vi "Display Features.vi"(6 "Local Data in":T2, 7 "UI References":T1, 8 "error in (no error)":errorcluster, 10 "Action":enum16{"All", "Preview", "Image"}(ring)=enum."Image") -> (0 "error out":errorcluster, 4 "Local Data out":T2)   [LabVIEW 2024]
uses:
  Controls/RVHR - Local Data.ctl
  Controls/Test Cluster.ctl
  Controls/Excluded Information.ctl
  Controls/Language.ctl
  Controls/Device_Type.ctl
  <vilib>/Utility/miscctls.llb/LVRectTypeDef.ctl
  <vilib>/Utility/miscctls.llb/LVBoundsTypeDef.ctl
  Controls/RVHR - UI Refs.ctl
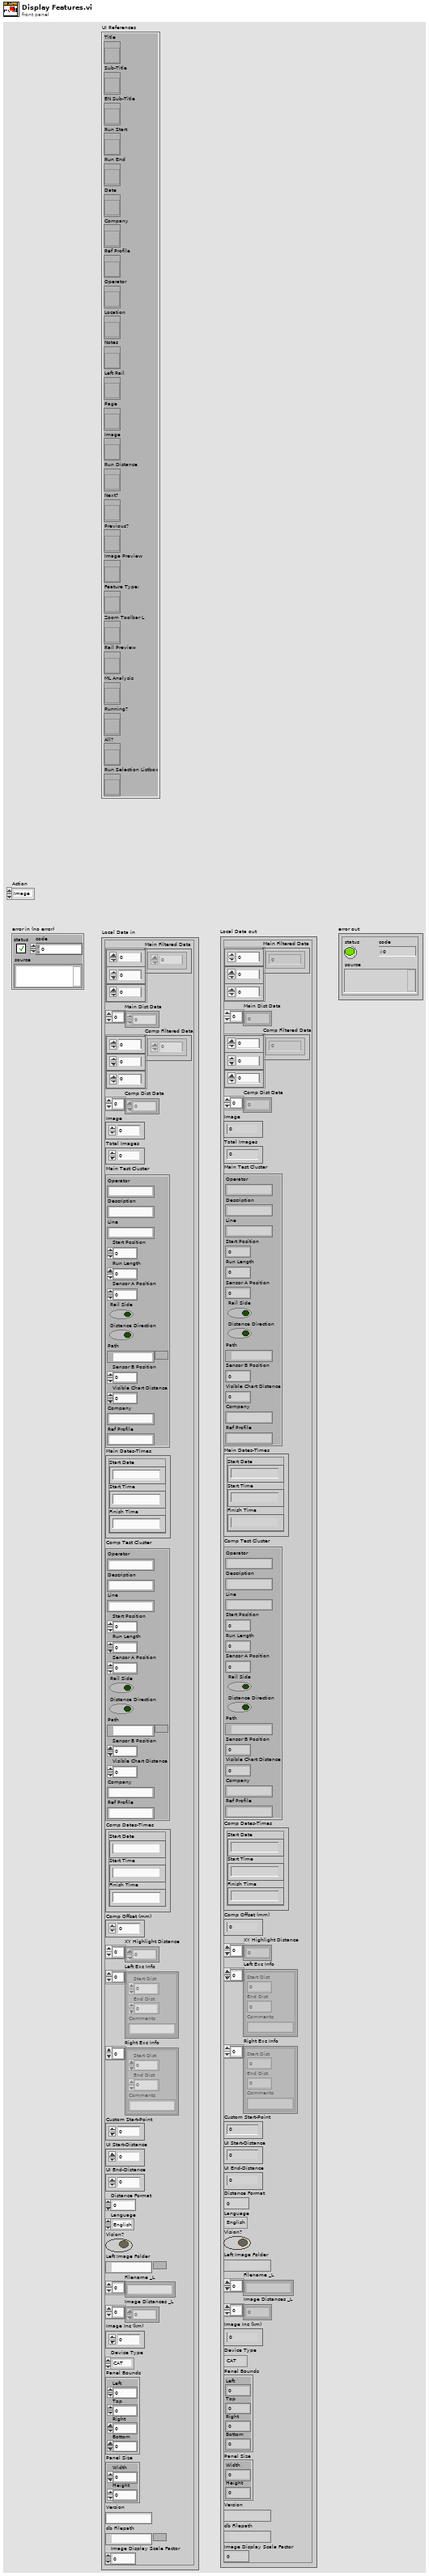
[diagram p1: front panel]
types:
  T1 = typedef "RVHR - UI Refs.ctl" = cluster{"Title":refnum<vi>, "Sub-Title":refnum<vi>, "EN Sub-Title":refnum<vi>, "Run Start":refnum<vi>, "Run End":refnum<vi>, "Date":refnum<vi>, "Company":refnum<vi>, "Ref Profile":refnum<vi>, "Operator":refnum<vi>, "Location":refnum<vi>, "Notes":refnum<vi>, "Left Rail":refnum<vi>, "Page":refnum<vi>, "Image":refnum<vi>, "Run Distance":refnum<vi>, "Next?":refnum<vi>, "Previous?":refnum<vi>, "Image Preview":refnum<vi>, "Feature Type:":refnum<vi>, "Zoom Toolbar L":refnum<vi>, "Rail Preview":refnum<vi>, "ML Analysis":refnum<vi>, "Running?":refnum<vi>, "All?":refnum<vi>, "Run Selection Listbox":refnum<vi>}
  T2 = typedef "RVHR - Local Data.ctl" = cluster{"Main Filtered Data":dbl[][][], "Main Dist Data":dbl[], "Comp Filtered Data":dbl[][][], "Comp Dist Data":dbl[], "Image":u16, "Total Images":u16, "Main Test Cluster":T3, "Main Dates-Times":cluster{"Start Date":string, "Start Time":string, "Finish Time":string}, "Comp Test Cluster":T3, "Comp Dates-Times":cluster{"Start Date":string, "Start Time":string, "Finish Time":string}, "Comp Offset (mm)":i64, "XY Highlight Distance":dbl[], "Left Exc Info":T4[], "Right Exc Info":T4[], "Custom Start-Point":dbl, "UI Start-Distance":dbl, "UI End-Distance":dbl, "Distance Format":u8, "Language":T5, "Vision?":bool, "Left Image Folder":path, "Filename _L":string[], "Image Distances _L":dbl[], "Image Inc (km)":dbl, "Device Type":T6, "Panel Bounds":T7, "Panel Size":T8, "Version":string, "db Filepath":path, "Image Display Scale Factor":dbl}
  T3 = typedef "Test Cluster.ctl" = cluster{"Operator":string, "Description":string, "Line":string, "Start Position":dbl, "Run Length":dbl, "Sensor A Position":dbl, "Rail Side":bool, "Distance Direction":bool, "Path":path, "Sensor B Position":dbl, "Visible Chart Distance":dbl, "Company":string, "Ref Profile":string}
  T4 = typedef "Excluded Information.ctl" = cluster{"Start Dist":dbl, "End Dist":dbl, "Comments":string}
  T5 = typedef "Language.ctl" = enum16{"English", "Chinese", "German"}
  T6 = typedef "Device_Type.ctl" = enum16{"CAT", "Bi-CAT", "YRCA", "RCA", "RV-HR", "TV-HR"}
  T7 = typedef "LVRectTypeDef.ctl" = cluster{"Left":i16, "Top":i16, "Right":i16, "Bottom":i16}
  T8 = typedef "LVBoundsTypeDef.ctl" = cluster{"Width":u32, "Height":u32}
  T9 = enum16{"Get Image", "Get Preview", "Add", "Remove"}
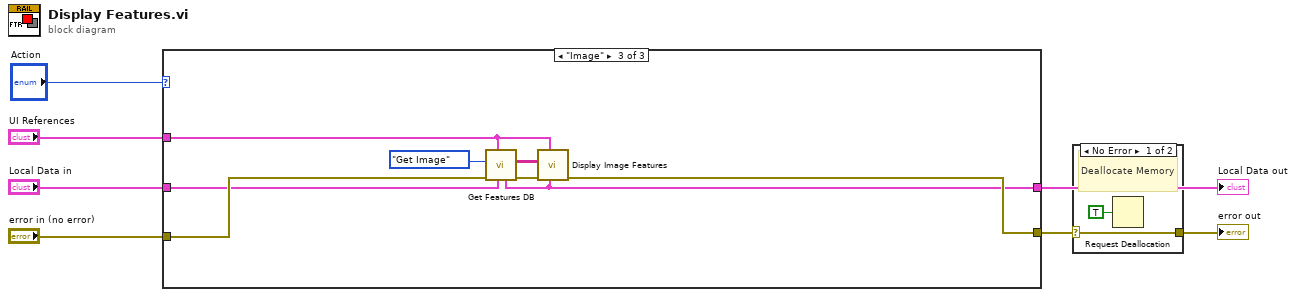
[diagram p0: block diagram]
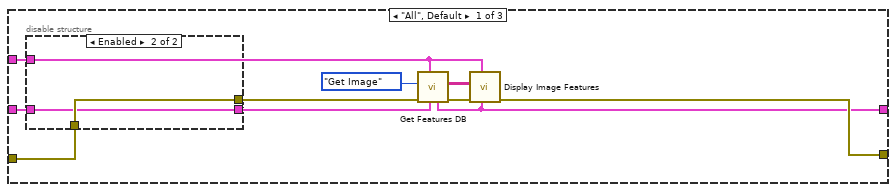
[diagram p3: hidden frame]
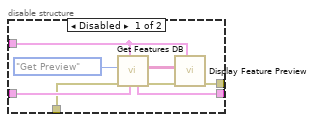
[diagram p4: hidden frame]
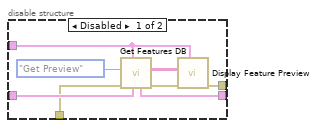
[diagram p6: hidden frame]
diagram:
  n1 = case shown="\"Image\"" "Action" {
    tunnel: "Local Data in" -> [w12 w32 w45]
    tunnel: [w8 w29 w43] -> w6
    tunnel: [w9 w28 w44] -> w2
    tunnel: "error in (no error)" -> [w11 w31 w46]
    tunnel: "UI References" -> [w10 w30 w47]
    frame "All", Default {
      n2 = disable-structure shown="Enabled" {
        disable-tunnel: [w24 w27] -> w17
        disable-tunnel: [w22 w26] -> w14
        disable-tunnel: w12 -> [w20 w26]
        disable-tunnel: w11 -> [w19 w27]
        disable-tunnel: w10 -> [w18 _]
        frame Disabled {
          n3 = call "Get Features DB.vi"("Local Data in"=w20, "UI References"=w18, "error in (no error)"=w19, "Action"=T9."Get Preview") -> ("error out"=w25:errorcluster, "Features"=w23:string[][], "Local Data out"=w22:T2)  [unwired: 3 in, 2 out]
          n4 = call "Display Feature Preview.vi"("UI References"=w18, "error in (no error)"=w25, "Features"=w23) -> ("error out"=w24:errorcluster)  [unwired: 8 in]
        }
        frame Enabled {
        }
      }
      n5 = call "Get Features DB.vi"("Local Data in"=w14, "UI References"=w10, "error in (no error)"=w17, "Action"=T9."Get Image") -> ("error out"=w16:errorcluster, "Features"=w15:string[][], "Local Data out"=w8:T2)  [unwired: 3 in, 2 out]
      n6 = call "Display Image Features.vi"("Local Data"=w8, "UI References"=w10, "error in (no error)"=w16, "Features"=w15) -> ("error out"=w9:errorcluster)  [unwired: 7 in]
    }
    frame "Preview" {
      n7 = disable-structure shown="Enabled" {
        disable-tunnel: w32 -> [w37 w41]
        disable-tunnel: w31 -> [w36 w42]
        disable-tunnel: w30 -> [w35 _]
        disable-tunnel: [w34 w41] -> w29
        disable-tunnel: [w33 w42] -> w28
        frame Disabled {
          n8 = call "Get Features DB.vi"("Local Data in"=w37, "UI References"=w35, "error in (no error)"=w36, "Action"=T9."Get Preview") -> ("error out"=w40:errorcluster, "Features"=w39:string[][], "Local Data out"=w34:T2)  [unwired: 3 in, 2 out]
          n9 = call "Display Feature Preview.vi"("UI References"=w35, "error in (no error)"=w40, "Features"=w39) -> ("error out"=w33:errorcluster)  [unwired: 8 in]
        }
        frame Enabled {
        }
      }
    }
    frame "Image" {
      n10 = call "Get Features DB.vi"("Local Data in"=w45, "UI References"=w47, "error in (no error)"=w46, "Action"=T9."Get Image") -> ("error out"=w50:errorcluster, "Features"=w49:string[][], "Local Data out"=w43:T2)  [unwired: 3 in, 2 out]
      n11 = call "Display Image Features.vi"("Local Data"=w43, "UI References"=w47, "error in (no error)"=w50, "Features"=w49) -> ("error out"=w44:errorcluster)  [unwired: 7 in]
    }
  }
  "Local Data out" <- w6
  n12 = case shown="No Error" w2 {
    selector: w2 -> [w51 w53]
    tunnel: [w51 w53] -> w1
    frame No Error {
      # "Deallocate Memory"
      n13 = Request Deallocation(TRUE ("flag")) -> ()
    }
    frame Error {
    }
  }
  "error out" <- w1
